vi "Orca Flash Capture File Name Increment.vi"(0 "Path In":path, 9 "Cycle":u16, 11 "Step":u16) -> (4 "Path Out":path)   [LabVIEW 2020]
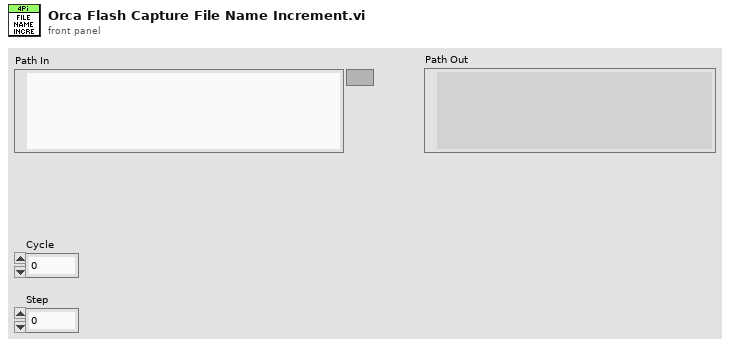
[diagram p1: front panel]
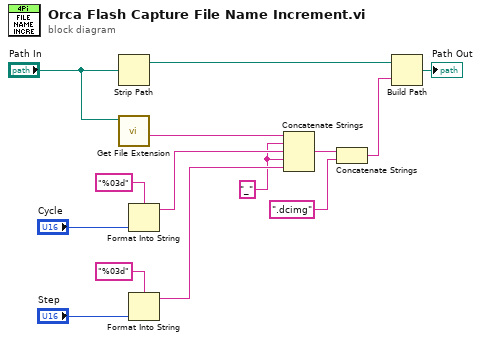
[diagram p0: block diagram]
diagram:
  w6 = "_"
  n1 = Strip Path(path="Path In") -> (stripped path=w5:path)  [unwired: 1 out]
  n2 = call <vilib>:"Get File Extension.vi"("file"="Path In") -> ("filename without extension"=w7:string)  [unwired: 6 in, 4 out]
  n3 = Format Into String(format string="%03d", "Cycle") -> (resulting string=w10:string)  [unwired: 2 in, 1 out]
  n4 = Format Into String(format string="%03d", "Step") -> (resulting string=w9:string)  [unwired: 2 in, 1 out]
  n5 = Concatenate Strings(w7, w6, w10, w6, w9) -> (w4:string)
  n6 = Concatenate Strings(w4, ".dcimg") -> (w2:string)
  n7 = Build Path(base path=w5, name or relative path=w2) -> (appended path=→"Path Out":path)
